vi "test_CCDSetAndGetSignalOut.vi"(6 "Delay between send and receive [ms]":i32=100, 7 "Test should pass":bool=TRUE, 8 "error in":errorcluster, 9 "tear down connection":bool=TRUE, 10 "set-up a connection":bool=TRUE, 11 "device selection":enum16{"monochromator", "CCD", "SCD"}(ring)=enum."CCD") -> (0 "error out":errorcluster)   [LabVIEW 2023]
uses:
  Classes/CCD/CCD.lvclass
  <vilib>/addons/_JKI Toolkits/Caraya/classes/Assert/Assert Equal Value and Type_Variant.vi
  <vilib>/addons/_JKI Toolkits/Caraya/classes/Assert/Assert Not Error.vi
  <vilib>/addons/_JKI Toolkits/Caraya/classes/Test/Test.lvclass
  <vilib>/addons/_JKI Toolkits/Caraya/classes/Assert/Assert.lvclass
  C:/Users/grju/Desktop/AbgelegteDokumente/Kunden/Horiba/horiba-labview-sdk/Source/Classes/GenericDevice/GenericDevice.lvclass
  C:/Users/grju/Desktop/AbgelegteDokumente/Kunden/Horiba/horiba-labview-sdk/Source/Classes/CCD/CCD.lvclass
panel:
  # "Connector Pane"
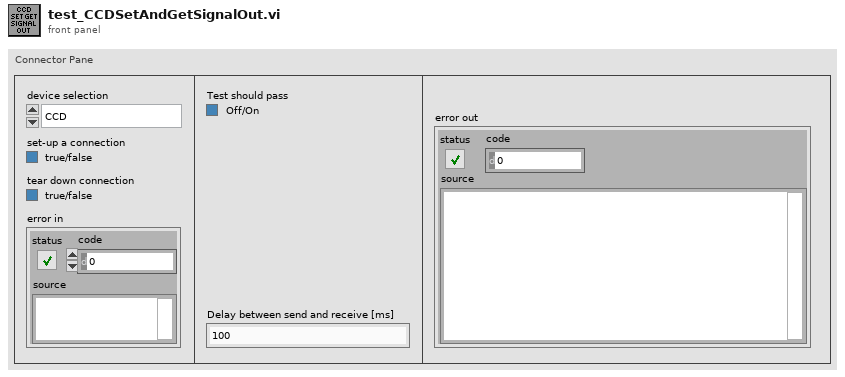
[diagram p1: front panel]
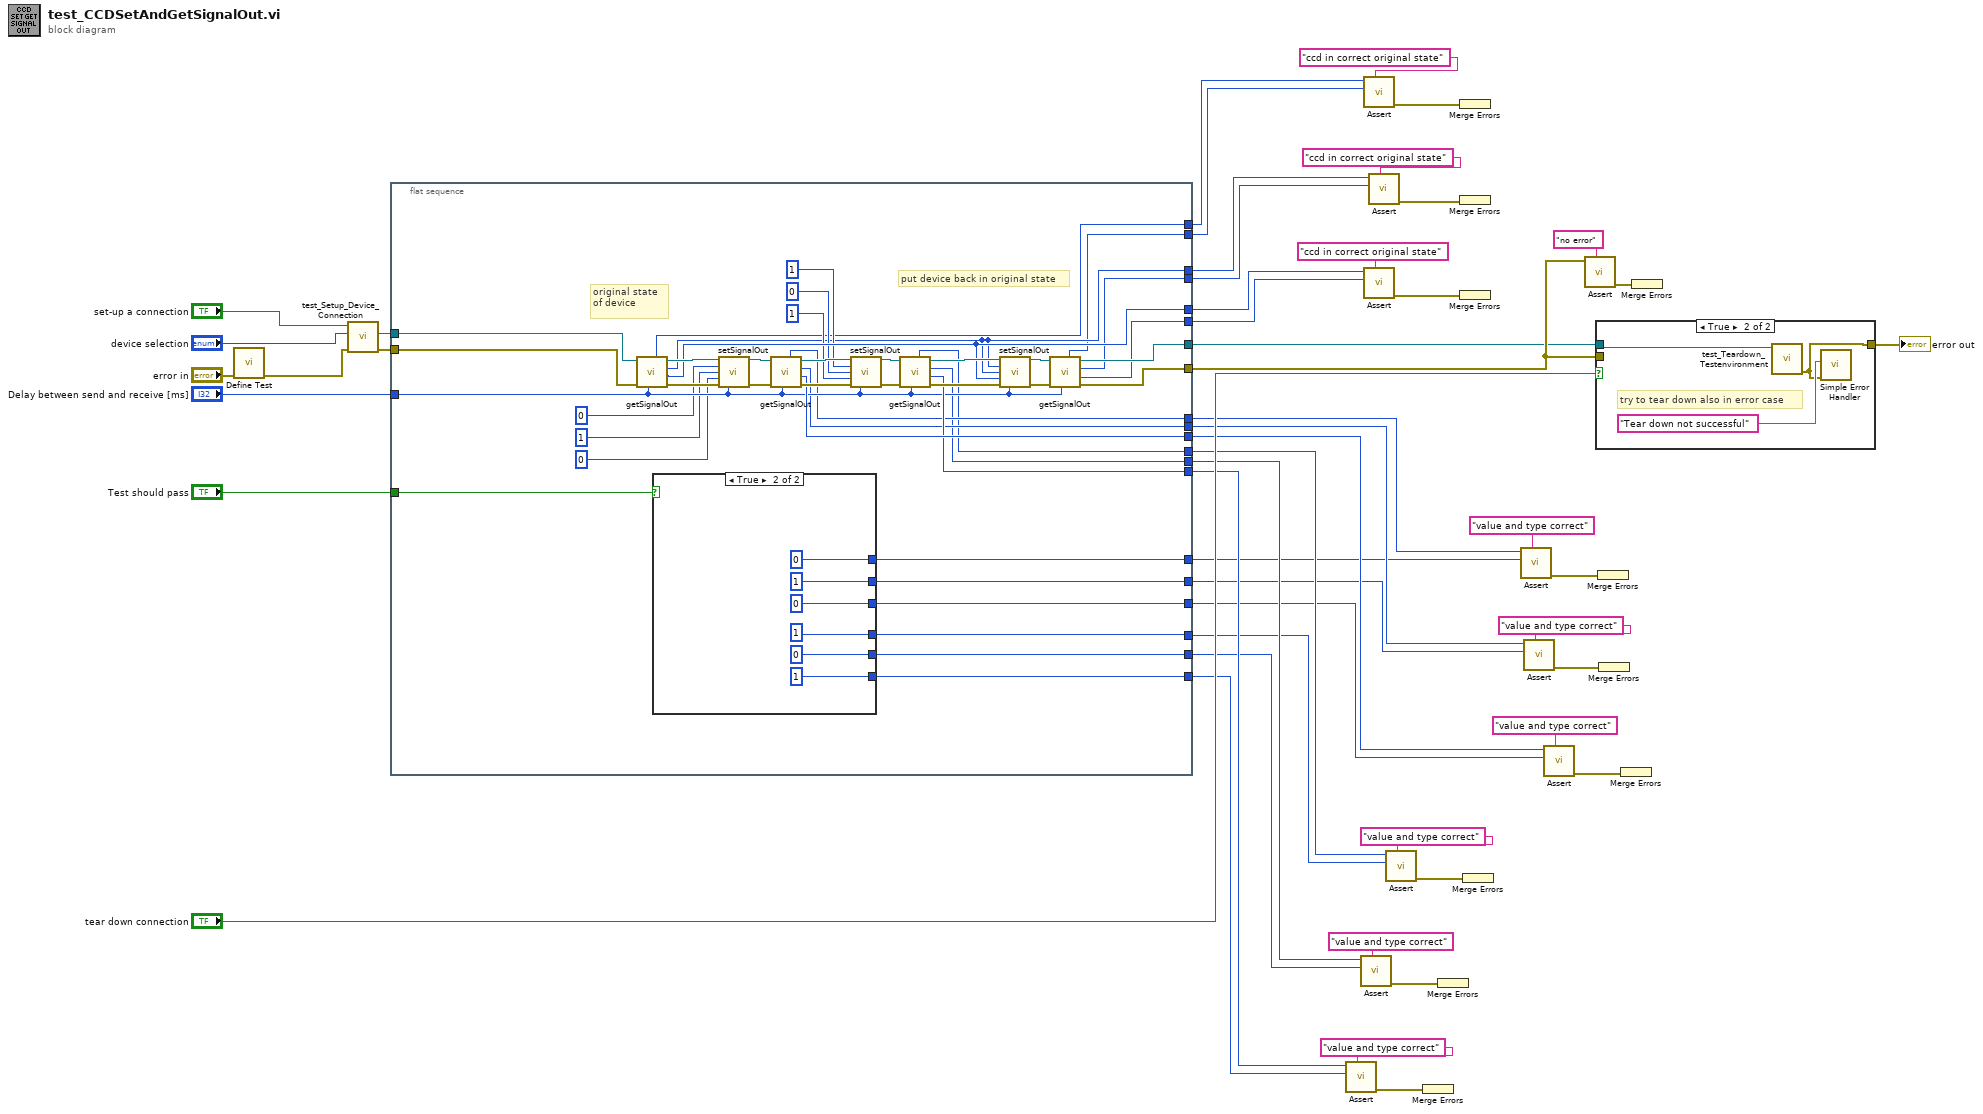
[diagram p0: block diagram]
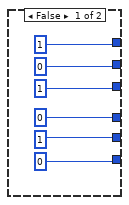
[diagram p2: hidden frame]
diagram:
  n1 = call <vilib>:"Define Test.vi"("error in (no error)"="error in") -> ("error out"=w28:errorcluster)  [unwired: 9 in, 1 out]
  n2 = call "test_Setup_Device_Connection.vi"("error in (no error)"=w28, "device selection"="device selection", "set-up a connection"="set-up a connection") -> ("error out"=w29:errorcluster, "CCD.lvclass"=w27:refnum<class "CCD.lvclass">)  [unwired: 5 in, 2 out]
  n3 = flat-sequence {
    tunnel: w29 -> [w90]
    tunnel: w27 -> [w91]
    tunnel: [w76] -> w42
    tunnel: "Test should pass" -> [w92]
    tunnel: [w77] -> w41
    tunnel: [w54] -> w40
    tunnel: [w56] -> w9
    tunnel: [w68] -> w37
    tunnel: [w69] -> w36
    tunnel: [w75] -> w8
    tunnel: [w74] -> w30
    tunnel: [w55] -> w10
    tunnel: [w53] -> w7
    tunnel: "Delay between send and receive [ms]" -> [w73]
    tunnel: [w51] -> w23
    tunnel: [w57] -> w22
    tunnel: [w52] -> w21
    tunnel: [w58] -> w20
    tunnel: [w64] -> w6
    tunnel: [w63] -> w5
    tunnel: [w62] -> w4
    tunnel: [w61] -> w3
    tunnel: [w60] -> w2
    tunnel: [w59] -> w1
    frame #0 {
      # "put device back in original state"
      # "original state of device"
      n4 = call "getSignalOut.vi"("Delay between send and receive [ms]"=w73, "error in (no error)"=w90, "CCD in"=w91) -> ("error out"=w88:errorcluster, "signalType"=w68:i32, "event"=w57:i32, "CCD out"=w89:refnum<class "CCD.lvclass">, "address"=w58:i32)  [unwired: 4 in]
      n5 = case shown="True" w92 {
        tunnel: [1 ("exposure time [ms]") 0 ("token")] -> w64
        tunnel: [0 ("exposure time [ms]") 1 ("token")] -> w63
        tunnel: [1 ("exposure time [ms]") 0 ("token")] -> w62
        tunnel: [0 ("token") 1 ("exposure time [ms]")] -> w61
        tunnel: [1 ("token") 0 ("exposure time [ms]")] -> w60
        tunnel: [0 ("token") 1 ("exposure time [ms]")] -> w59
        frame False {
        }
        frame True {
        }
      }
      n6 = call "setSignalOut.vi"("CCD in"=w89, "address"=0 ("token"), "event"=1 ("token"), "signalType"=0 ("token"), "error in (no error)"=w88, "Delay between send and receive [ms]"=w73) -> ("CCD out"=w86:refnum<class "CCD.lvclass">, "error out"=w87:errorcluster)  [unwired: 6 in, 2 out]
      n7 = call "getSignalOut.vi"("Delay between send and receive [ms]"=w73, "error in (no error)"=w87, "CCD in"=w86) -> ("error out"=w82:errorcluster, "signalType"=w75:i32, "event"=w56:i32, "CCD out"=w83:refnum<class "CCD.lvclass">, "address"=w55:i32)  [unwired: 4 in]
      n8 = call "setSignalOut.vi"("CCD in"=w83, "address"=1 ("exposure time [ms]"), "event"=0 ("exposure time [ms]"), "signalType"=1 ("exposure time [ms]"), "error in (no error)"=w82, "Delay between send and receive [ms]"=w73) -> ("CCD out"=w84:refnum<class "CCD.lvclass">, "error out"=w85:errorcluster)  [unwired: 6 in, 2 out]
      n9 = call "getSignalOut.vi"("Delay between send and receive [ms]"=w73, "error in (no error)"=w85, "CCD in"=w84) -> ("error out"=w79:errorcluster, "signalType"=w74:i32, "event"=w54:i32, "CCD out"=w80:refnum<class "CCD.lvclass">, "address"=w53:i32)  [unwired: 4 in]
      n10 = call "setSignalOut.vi"("CCD in"=w80, "address"=w57, "event"=w57, "signalType"=w68, "error in (no error)"=w79, "Delay between send and receive [ms]"=w73) -> ("CCD out"=w78:refnum<class "CCD.lvclass">, "error out"=w81:errorcluster)  [unwired: 6 in, 2 out]
      n11 = call "getSignalOut.vi"("Delay between send and receive [ms]"=w73, "error in (no error)"=w81, "CCD in"=w78) -> ("error out"=w76:errorcluster, "signalType"=w69:i32, "event"=w51:i32, "CCD out"=w77:refnum<class "CCD.lvclass">, "address"=w52:i32)  [unwired: 4 in]
    }
  }
  n12 = call-poly <vilib>:"Assert.vi"("Label"="value and type correct" ("Label (VI Title)"), "Y"=w1, "X"=w30) -> ("error out"=w32:errorcluster)  [unwired: 7 in, 1 out]
  n13 = call-poly <vilib>:"Assert.vi"("Label"="value and type correct" ("Label (VI Title)"), "Y"=w2, "X"=w40) -> ("error out"=w49:errorcluster)  [unwired: 7 in, 1 out]
  n14 = call-poly <vilib>:"Assert.vi"("Label"="ccd in correct original state" ("Label (VI Title)"), "Y"=w21, "X"=w20) -> ("error out"=w19:errorcluster)  [unwired: 7 in, 1 out]
  n15 = call-poly <vilib>:"Assert.vi"("Label"="ccd in correct original state" ("Label (VI Title)"), "Y"=w36, "X"=w37) -> ("error out"=w39:errorcluster)  [unwired: 7 in, 1 out]
  n16 = call-poly <vilib>:"Assert.vi"("Label"="ccd in correct original state" ("Label (VI Title)"), "Y"=w23, "X"=w22) -> ("error out"=w18:errorcluster)  [unwired: 7 in, 1 out]
  n17 = call-poly <vilib>:"Assert.vi"("Label"="value and type correct" ("Label (VI Title)"), "Y"=w3, "X"=w7) -> ("error out"=w12:errorcluster)  [unwired: 7 in, 1 out]
  n18 = Merge Errors(w32) -> ()  [unwired: 1 out]
  n19 = Merge Errors(w49) -> ()  [unwired: 1 out]
  n20 = Merge Errors(w19) -> ()  [unwired: 1 out]
  n21 = Merge Errors(w18) -> ()  [unwired: 1 out]
  n22 = Merge Errors(w39) -> ()  [unwired: 1 out]
  n23 = Merge Errors(w12) -> ()  [unwired: 1 out]
  n24 = call-poly <vilib>:"Assert.vi"("Label"="value and type correct" ("Label (VI Title)"), "Y"=w6, "X"=w10) -> ("error out"=w33:errorcluster)  [unwired: 7 in, 1 out]
  n25 = call-poly <vilib>:"Assert.vi"("Label"="value and type correct" ("Label (VI Title)"), "Y"=w5, "X"=w9) -> ("error out"=w17:errorcluster)  [unwired: 7 in, 1 out]
  n26 = call-poly <vilib>:"Assert.vi"("Label"="value and type correct" ("Label (VI Title)"), "Y"=w4, "X"=w8) -> ("error out"=w48:errorcluster)  [unwired: 7 in, 1 out]
  n27 = call-poly <vilib>:"Assert.vi"("Label"="no error" ("Label (VI Title)"), "Not Error?"=w42) -> ("error out"=w44:errorcluster)  [unwired: 8 in, 1 out]
  n28 = case shown="True" "tear down connection" {
    tunnel: w41 -> [_ w107]
    tunnel: [w105 w106] -> w35
    tunnel: w42 -> [w105 _]
    frame False {
    }
    frame True {
      # "try to tear down also in error case"
      n29 = call "test_Teardown_Testenvironment.vi"("GenericDevice.lvclass"=w107) -> ("error out"=w106:errorcluster)  [unwired: 9 in, 1 out]
      n30 = call <vilib>:"Simple Error Handler.vi"("error source (\" \")"="Tear down not successful" ("error source (\" \")"), "error in (no error)"=w106) -> ()  [unwired: 3 in, 5 out]
    }
  }
  "error out" <- w35
  n31 = Merge Errors(w33) -> ()  [unwired: 1 out]
  n32 = Merge Errors(w17) -> ()  [unwired: 1 out]
  n33 = Merge Errors(w48) -> ()  [unwired: 1 out]
  n34 = Merge Errors(w44) -> ()  [unwired: 1 out]
